vi "Compilation Message to String.vi"(4 "Message":T1) -> (1 "Messgae":string)   [LabVIEW 2016]
uses:
  Validate_message.ctl
  Validate_MessageStatus.ctl
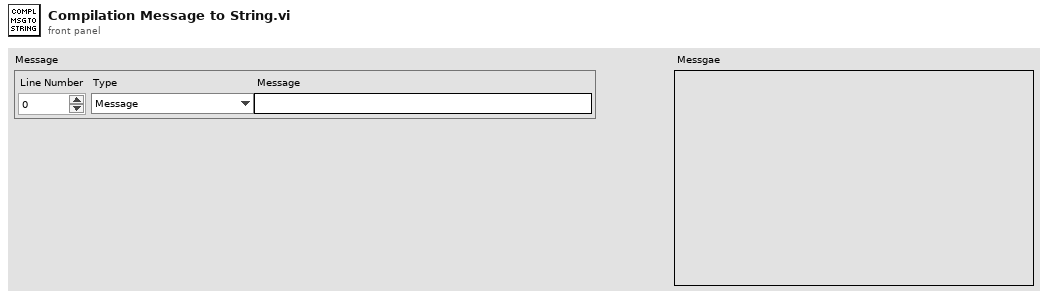
[diagram p1: front panel]
types:
  T1 = typedef "Validate_message.ctl" = cluster{"Line Number":i64, "Type":T2, "Message":string}
  T2 = typedef "Validate_MessageStatus.ctl" = enum16{"Message", "Warning", "Error"}
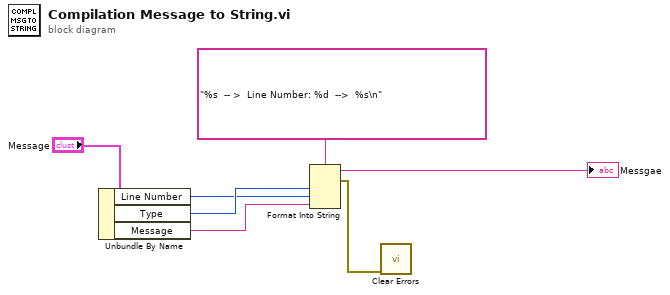
[diagram p0: block diagram]
diagram:
  n1 = Unbundle By Name("Message") -> ("Line Number"=w5:i64, "Type"=w6:T2, "Message"=w4:string)
  n2 = Format Into String(format string="%s  -- >  Line Number: %d  -->  %s\n", w6, w5, w4) -> (resulting string=→"Messgae":string, error out=w3:errorcluster)  [unwired: 2 in]
  n3 = call <vilib>:"Clear Errors.vi"("error in (no error)"=w3) -> ()  [unwired: 5 in, 2 out]
